vi "Load Configuration.vi"(8 "error in (no error)":errorcluster, 11 "hdl":i32) -> (0 "error out":errorcluster, 3 "hdl out":i32)   [LabVIEW 2013, in "Thorlabs_SC10.lvlib"]
doc: "cycle=n,\nThe CYCLE parameters (STOP temp, RAMP time, and HOLD time) can be programmed from the command line\ninterface as follows:\n1. Set the Step number to which the three parameters will apply by typing cycle=n, where n represents the\nStep number (1 to 5).\n2. Enter valid values for the STOP temp by typing stop=nnn.n (20.0 to 200.0 or TMAX)\n3. Enter valid values for the RAMP time by typing ramp=nnn (1 to 999)\n4. Enter valid values for the HOLD time by typing hold=nnn (1 to 999)\nUntil the CYCLE number is changed to another value, any values entered for STOP, RAMP, or HOLD will apply to\nthe current value of CYCLE."
uses:
  <instrlib>/Thorlabs_SC10/Thorlabs_SC10.lvlib
  <instrlib>/Thorlabs_SC10/Data/SC10CommandLib_x64.dll
  <instrlib>/Thorlabs_SC10/Data/SC10CommandLib_win32.dll
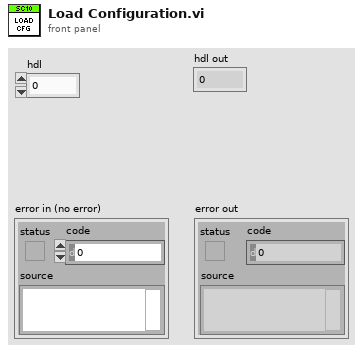
[diagram p1: front panel]
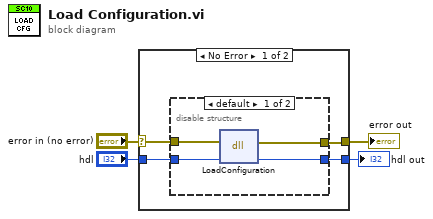
[diagram p0: block diagram]
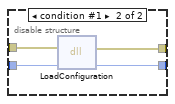
[diagram p2: hidden frame]
diagram:
  n1 = case shown="No Error" "error in (no error)" {
    selector: "error in (no error)" -> [w8 w17]
    tunnel: [w6 w17] -> w4
    tunnel: "hdl" -> [w7 _]
    tunnel: [w5 _] -> w1
    frame No Error {
      n2 = disable-structure shown="default" {
        disable-tunnel: w8 -> [w12 w16]
        disable-tunnel: w7 -> [w11 w15]
        disable-tunnel: [w10 w14] -> w6
        disable-tunnel: [w9 w13] -> w5
        frame condition #0 (active) {
          n3 = dll-call lib="C:/Program Files (x86)/National Instruments/LabVIEW 2013/instr.lib/Thorlabs_SC10/Data/SC10CommandLib_win32.dll" fn="LoadConfiguration"(error in=w12, "hdl"=w11) -> (error out=w10:errorcluster, "hdl"=w9:i32)  [unwired: 3 in, 1 out]
        }
        frame condition #1 {
          n4 = dll-call lib="C:/Program Files/National Instruments/LabVIEW 2013/instr.lib/Thorlabs_SC10/Data/SC10CommandLib_x64.dll" fn="LoadConfiguration"(error in=w16, "hdl"=w15) -> (error out=w14:errorcluster, "hdl"=w13:i32)  [unwired: 3 in, 1 out]
        }
      }
    }
    frame Error {
    }
  }
  "error out" <- w4
  "hdl out" <- w1
